vi "Configure Offset Compensation.vi"(6 "Offset Compensate Mode(2: Auto)":i32(ring)=2 items=["Disabled", "Enabled", "Auto"], 8 "error in (no error)":errorcluster, 9 "Channel List(\"\")":string, 10 "Function (5: 4-wire resistance)":i32(ring)=5 items=["4-wire Resistance"=5, "Temperature"=8], 11 "VISA resource name":refnum<visa-resource-name>) -> (0 "error out":errorcluster, 3 "VISA resource name out":refnum<visa-resource-name>)   [LabVIEW 2020, in "Keithley DMM6500 DAQ6500 Series.lvlib"]
doc: "Enables or disable offset compensation."
uses:
  <instrlib>/Keithley DMM6500 DAQ6500 Series/Keithley DMM6500 DAQ6500 Series.lvlib
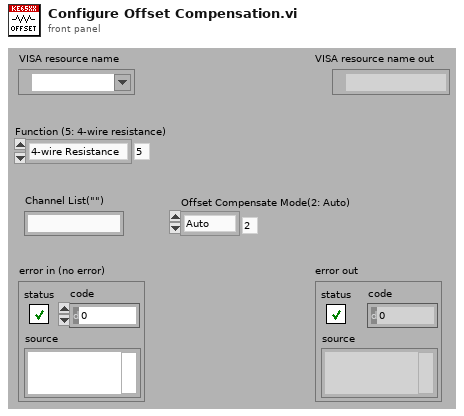
[diagram p1: front panel]
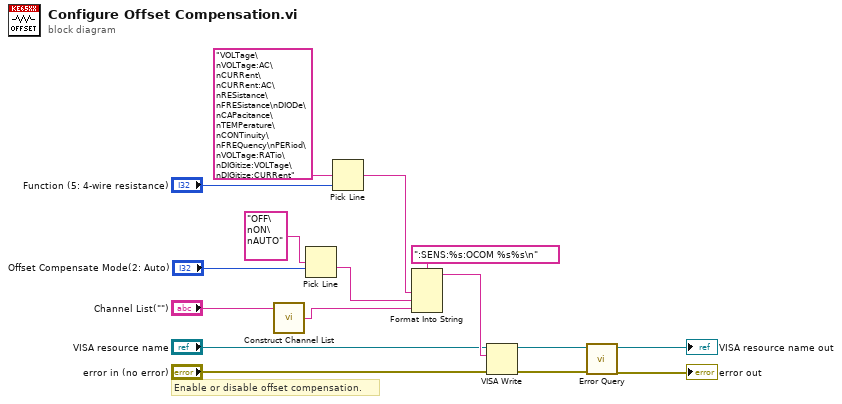
[diagram p0: block diagram]
diagram:
  # "Enable or disable offset compensation."
  n1 = call <instrlib>:"Construct Channel List.vi"("Channel List"="Channel List(\"\")") -> ("Channel List String"=w4:string)  [unwired: 2 in]
  n2 = Pick Line(multi-line string="OFF\nON\nAUTO", line index="Offset Compensate Mode(2: Auto)") -> (output string=w3:string)  [unwired: 1 in]
  n3 = Pick Line(multi-line string="VOLTage\nVOLTage:AC\nCURRent\nCURRent:AC\nRESistance\nFRESistance\nDIODe\nCAPacitance\nTEMPerature\nCONTinuity\nFREQuency\nPERiod\nVOLTage:RATio\nDIGitize:VOLTage\nDIGitize:CURRent", line index="Function (5: 4-wire resistance)") -> (output string=w7:string)  [unwired: 1 in]
  n4 = Format Into String(format string=":SENS:%s:OCOM %s%s\n", w7, w3, w4) -> (resulting string=w15:string)  [unwired: 2 in, 1 out]
  n5 = VISA Write(VISA resource name="VISA resource name", write buffer=w15, error in (no error)="error in (no error)") -> (VISA resource name out=w12:refnum<visa-resource-name>, error out=w11:errorcluster)  [unwired: 1 out]
  n6 = call <instrlib>:"Error Query.vi"("error in (no error)"=w11, "VISA resource name"=w12) -> ("error out"=→"error out":errorcluster, "VISA resource name out"=→"VISA resource name out":refnum<visa-resource-name>)  [unwired: 6 in, 2 out]
